vi "InvFilter-Create Spectrum.vi"(0 "Calibration file":path, 1 "Fmin (Hz)":dbl=1000.0, 2 "Fmax (Hz)":dbl=inf, 5 "Fs (Hz)":dbl=100000.0, 7 "Npts":i32=2, 9 "Brickwall (T)":bool=TRUE, 11 "error in (no error)":errorcluster) -> (4 "Interp Freq (Hz)":dbl[](array[numeric]), 6 "Magnitude (dB)":dbl[](array[numeric]), 8 "Phase (degrees)":dbl[](array[numeric]), 10 "reference":dbl, 15 "error out":errorcluster)   [LabVIEW 2020]
uses:
  epl-vi-lib/Signal Synthesis VIs/Controls/Advanced Filter XCtl/Filter Data.ctl
  epl-vi-lib/Signal Synthesis VIs/Filter VIs/Filter-Bandwidth Units.ctl
  epl-vi-lib/Utility VIs/Math VIs/Z to dB, degrees (1D).vi
  epl-vi-lib/Utility VIs/Math VIs/dB to Linear (1D).vi
  epl-vi-lib/Signal Synthesis VIs/Controls/Advanced Filter XCtl/Advanced Filter XCtl.xctl
panel:
  in  "Filter in":T1={"Type"=enum."Bandpass", "CF (kHz)"=0.0, "BW (kHz)"=0.0, "Cascade"=TRUE, "Quadrature"=FALSE, "Scale Factor"=0.0, "Stages"=[], "Class"=enum."Elliptic", "Order"=7, "BWUnits"=enum."Linear"} {"Stages"."IIR Filter"."Forward Coefficients" format="%.4f"; "Stages"."IIR Filter"."Reverse Coefficients" format="%.4f"}
  out "Calibration":T3(graph)
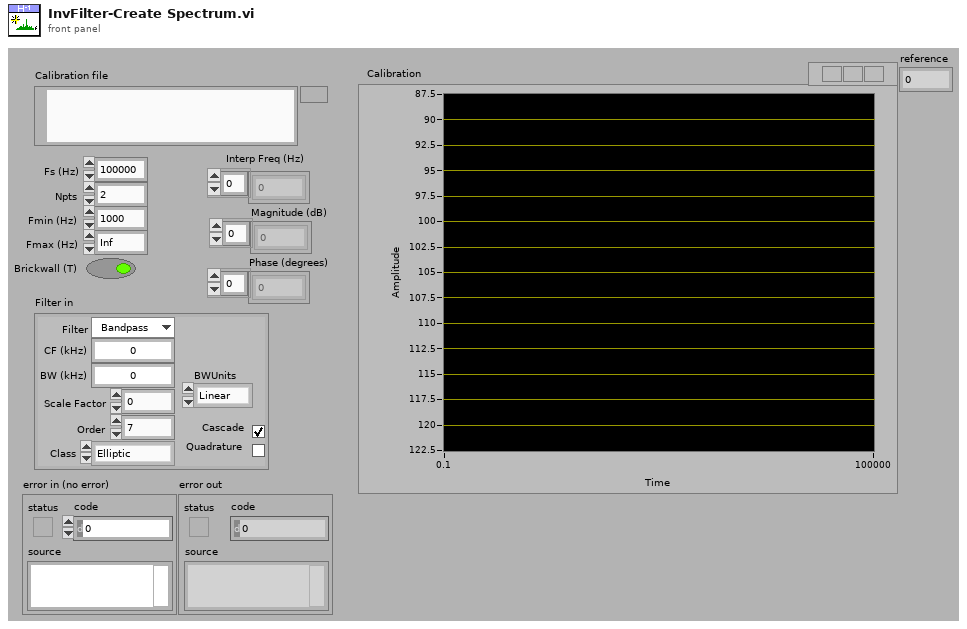
[diagram p1: front panel]
types:
  T1 = typedef "Advanced Filter XCtl.xctl/Filter Data.ctl" = cluster{"Type":enum16{"Lowpass", "Highpass", "Bandpass", "Bandstop", "OFF"}, "CF (kHz)":dbl, "BW (kHz)":dbl, "Cascade":bool, "Quadrature":bool, "Scale Factor":dbl, "Stages":cluster{"IIR Filter":cluster{"filter structure":enum32{"IIR 2nd Order", "IIR 4th Order"}, "Reverse Coefficients":dbl[], "Forward Coefficients":dbl[]}, "State":dbl[]}[], "Class":enum16{"Elliptic", "Butterworth"}, "Order":i32, "BWUnits":T2}
  T2 = typedef "Filter-Bandwidth Units.ctl" = enum16{"Linear", "Octaves", "Min-Max"}
  T3 = cluster{"Interp Freq (Hz)":dbl[], "Interp Magnitude (dB)":dbl[]}[]
  T4 = cluster{"Interp Freq (Hz)":dbl[], "Interp Magnitude (dB)":dbl[]}
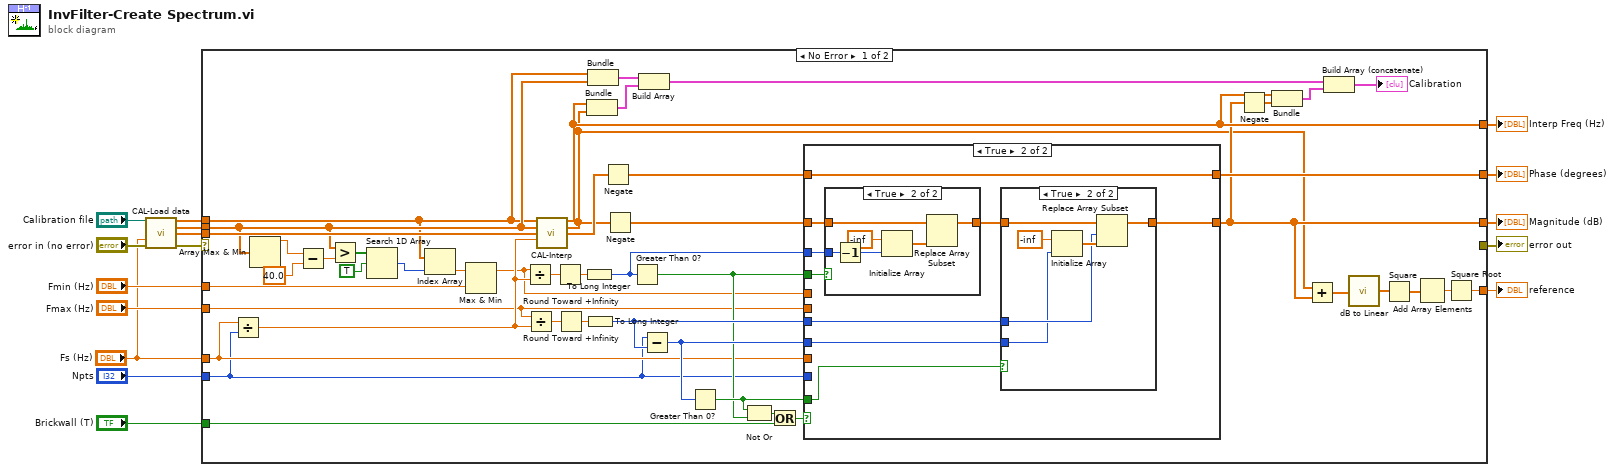
[diagram p0: block diagram]
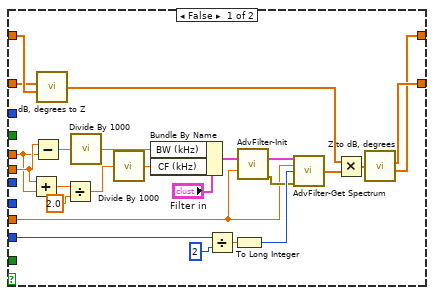
[diagram p2: hidden frame]
diagram:
  n1 = call "CAL-Load data.vi"("user path"="Calibration file", "Desired Fs (Hz)"="Fs (Hz)", "error in (no error)"="error in (no error)") -> ("Frequency (Hz)"=w15:dbl[], "Mag"=w13:dbl[], "Phase"=w12:dbl[], "error out"=w10:errorcluster)  [unwired: 5 in, 4 out]
  n2 = case shown="No Error" w10 {
    selector: w10 -> [_ w110]
    tunnel: "Fs (Hz)" -> [w41 _]
    tunnel: w15 -> [w28 _]
    tunnel: "Npts" -> [w40 _]
    tunnel: w13 -> [w34 _]
    tunnel: w12 -> [w62 _]
    tunnel: [_ w110] -> w9
    tunnel: "Fmin (Hz)" -> [w25 _]
    tunnel: "Fmax (Hz)" -> [w42 _]
    tunnel: [w23 _] -> w6
    tunnel: [w49 _] -> w5
    tunnel: [w39 _] -> w4
    tunnel: "Brickwall (T)" -> [w46 _]
    tunnel: [w17 _] -> w1
    frame No Error {
      n3 = Divide(x=w41, y=w40) -> (x/y=w50:dbl)
      n4 = Array Max & Min(array=w34) -> (max value=w33:dbl)  [unwired: 3 out]
      n5 = Subtract(x=w33, y=40.0) -> (x-y=w31:dbl)
      n6 = Greater?(x=w34, y=w31) -> (0:w30:bool[])
      n7 = Search 1D Array(1D array=w30, element=TRUE) -> (index of element=w27:i32)  [unwired: 1 in]
      n8 = Index Array(array=w28, index=w27) -> (element=w26:dbl)
      n9 = Max & Min(x=w26, y=w25) -> (max(x,y)=w24:dbl)  [unwired: 1 out]
      n10 = Divide(x=w24, y=w50) -> (x/y=w58:dbl)
      n11 = Divide(x=w42, y=w50) -> (x/y=w55:dbl)
      n12 = call "CAL-Interp.vi"("Frequency (Hz)"=w28, "Magnitude (dB)"=w34, "Phase (degrees)"=w62, "df (Hz)"=w50) -> ("Interp Freq (Hz)"=w39:dbl[], "Interp Magnitude (dB)"=w19:dbl[], "Interp Phase (degrees)"=w51:dbl[])  [unwired: 8 in, 1 out]
      n13 = Round Toward +Infinity(x=w58) -> (ceil(x): smallest int >= x=w57:dbl)
      n14 = Round Toward +Infinity(x=w55) -> (ceil(x): smallest int >= x=w54:dbl)
      n15 = To Long Integer(number=w57) -> (32bit integer=w56:i32)
      n16 = To Long Integer(number=w54) -> (32bit integer=w53:i32)
      n17 = Bundle("Interp Freq (Hz)"=w39, "Interp Magnitude (dB)"=w19) -> (w59:T4)  [unwired: 1 in]
      n18 = Bundle("Frequency (Hz)"=w28, "Mag"=w34) -> (w60:cluster{"Frequency (Hz)":dbl[], "Mag":dbl[]})  [unwired: 1 in]
      n19 = Negate(x=w51) -> (-x=w48:dbl[])
      n20 = Negate(x=w19) -> (-x=w61:dbl[])
      n21 = Greater Than 0?(x=w56) -> (x > 0?=w43:bool)
      n22 = Build Array(w60, w59) -> (w38:T3)
      n23 = Subtract(x=w40, y=w53) -> (x-y=w52:i32)
      n24 = Greater Than 0?(x=w52) -> (x > 0?=w44:bool)
      n25 = Not Or(1:w43, 2:w44) -> (0:w45:bool)
      n26 = Or(x=w45, y=w46) -> (x .or. y?=w47:bool)
      n27 = case shown="True" w47 {
        tunnel: w61 -> [w68 w95]
        tunnel: w43 -> [_ w94]
        tunnel: w56 -> [_ w93]
        tunnel: w44 -> [_ w91]
        tunnel: w53 -> [_ w90]
        tunnel: w52 -> [_ w89]
        tunnel: [w65 w88] -> w23
        tunnel: [w64 w87] -> w49
        tunnel: w48 -> [w69 w87]
        tunnel: w24 -> [w73 _]
        tunnel: w42 -> [w74 _]
        tunnel: w41 -> [w72 _]
        tunnel: w40 -> [w71 _]
        frame False {
          n28 = Add(x=w74, y=w73) -> (x+y=w75:dbl)
          n29 = Subtract(x=w74, y=w73) -> (x-y=w78:dbl)
          n30 = call "dB, degrees to Z.vi"("Magnitude (dB)"=w68, "Phase (degrees)"=w69) -> ("Z"=w67:cdb[])  [unwired: 5 in]
          n31 = Divide(x=w75, y=2.0) -> (x/y=w77:dbl)
          n32 = call "Divide By 1000.vi"("X"=w78) -> ("X/1000"=w82:dbl)
          n33 = call "Divide By 1000.vi"("X"=w77) -> ("X/1000"=w83:dbl)
          n34 = Bundle By Name(cluster="Filter in", "BW (kHz)"=w82, "CF (kHz)"=w83) -> (w79:T1)
          n35 = Divide(x=w71, y=2) -> (x/y=w85:dbl)
          n36 = To Long Integer(number=w85) -> (32bit integer=w86:i32)
          n37 = call "AdvFilter-Init.vi"("Filter"=w79, "Sampling rate (Hz)"=w72) -> ("Filter out"=w80:T1, "error out"=w81:errorcluster)  [unwired: 12 in]
          n38 = call "AdvFilter-Get Spectrum.vi"("Filter in"=w80, "Sampling Rate (Hz)"=w72, "Npts"=w86, "error in (no error)"=w81) -> ("spectrum"=w63:cdb[])  [unwired: 9 in, 2 out]
          n39 = Multiply(x=w67, y=w63) -> (x*y=w66:cdb[])
          n40 = call-poly "Z to dB, degrees.vi"("Z"=w66) -> ("Magnitude (dB)"=w65:dbl[], "Phase (degrees)"=w64:dbl[])  [unwired: 5 in]
        }
        frame True {
          n41 = case shown="True" w94 {
            tunnel: w95 -> [w103 w109]
            tunnel: [w103 w106] -> w92
            tunnel: w93 -> [_ w105]
            frame False {
            }
            frame True {
              n42 = Decrement(x=w105) -> (x-1=w104:i32)
              n43 = Initialize Array(-inf ("element"), w104) -> (w107:dbl[])
              n44 = Replace Array Subset(array=w109, new element=w107) -> (w106:dbl[])  [unwired: 1 in]
            }
          }
          n45 = case shown="True" w91 {
            tunnel: w92 -> [w96 w102]
            tunnel: [w96 w99] -> w88
            tunnel: w90 -> [_ w98]
            tunnel: w89 -> [_ w97]
            frame False {
            }
            frame True {
              n46 = Initialize Array(-inf ("element"), w97) -> (w100:dbl[])
              n47 = Replace Array Subset(array=w102, new element=w100, index=w98) -> (w99:dbl[])
            }
          }
        }
      }
      n48 = Negate(x=w23) -> (-x=w35:dbl[])
      n49 = Bundle("Interp Freq (Hz)"=w39, w35) -> (w37:cluster{"Interp Freq (Hz)":dbl[], dbl[]})  [unwired: 1 in]
      n50 = Add(x=w19, y=w23) -> (x+y=w20:dbl[])
      n51 = Build Array (concatenate)(w38, w37) -> (→"Calibration":T3)
      n52 = call-poly "dB to Linear.vi"("dB"=w20) -> ("linear"=w22:dbl[])
      n53 = Square(x=w22) -> (x^2=w21:dbl[])
      n54 = Add Array Elements(numeric array=w21) -> (sum=w18:dbl)
      n55 = Square Root(x=w18) -> (sqrt(x)=w17:dbl)
    }
    frame Error {
    }
  }
  "error out" <- w9
  "Magnitude (dB)" <- w6
  "Phase (degrees)" <- w5
  "Interp Freq (Hz)" <- w4
  "reference" <- w1
